vi "To Binary.vi"(8 "error in (no error)":errorcluster, 9 "byte order":T1(ring), 10 "Binary In":string, 11 "Double Float in":refnum<class "AbsFunc_One Term_DBL.lvclass">) -> (0 "error out":errorcluster, 2 "Binary":string, 3 "Double Float out":refnum<class "AbsFunc_One Term_DBL.lvclass">)   [LabVIEW 2021, in "AbsFunc_One Term_DBL.lvclass"]
uses:
  AbsFunc_One Term_DBL.lvclass
  AbsFunc_One Term_DBL.lvclass/AbsFunc_One Term_DBL.ctl
  Abs_Types/Double Float/Abs_Double Float.lvclass
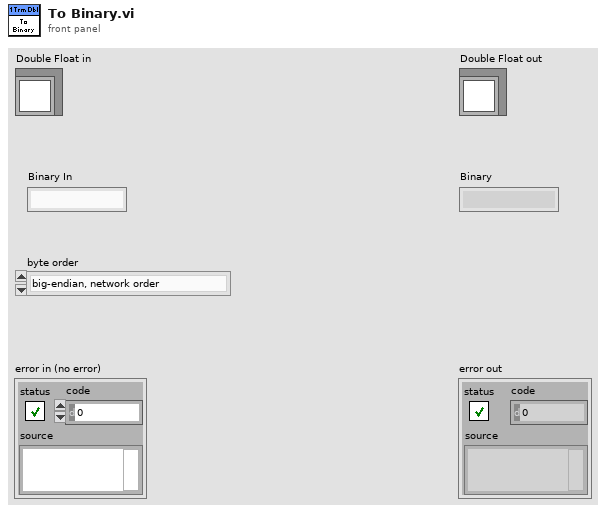
[diagram p1: front panel]
types:
  T1 = enum16{"big-endian, network order", "native, host order", "little-endian"}
  T2 = typedef "One Term_DBL.lvclass/Abstract Type.ctl" = refnum<class "Abs_Double Float.lvclass">
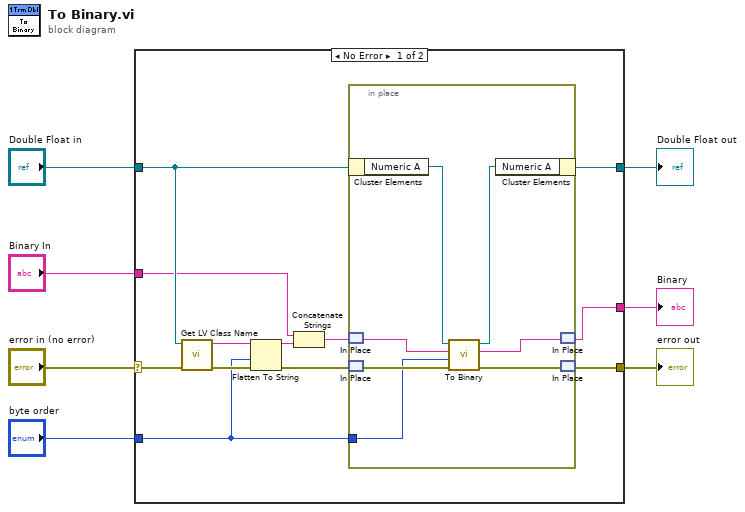
[diagram p0: block diagram]
diagram:
  n1 = case shown="No Error" "error in (no error)" {
    selector: "error in (no error)" -> [w19 w27]
    tunnel: "Binary In" -> [w10 w28]
    tunnel: "Double Float in" -> [w18 w29]
    tunnel: "byte order" -> [w12 _]
    tunnel: [w17 w27] -> w3
    tunnel: [w16 w28] -> w2
    tunnel: [w15 w29] -> w1
    frame No Error {
      n2 = call <vilib>:"Get LV Class Name.vi"("error in (no error)"=w19, "object"=w18) -> ("error out"=w13:errorcluster, "class name"=w14:string)  [unwired: 8 in]
      n3 = Flatten To String(anything=w14, byte order (0:big-endian, network order)=w12, error in (no error)=w13) -> (data string=w11:string, error out=w8:errorcluster)  [unwired: 1 in, 1 out]
      n4 = Concatenate Strings(w10, w11) -> (w9:string)
      n5 = in-place {
        in-place-border: w12 -> [w21]
        n6 = in-place-cluster #1(w18) -> ("Numeric A"=w26:T2)
        n7 = in-place-match #2(w9) -> (w24:string)
        n8 = in-place-match #3(w8) -> (w22:errorcluster)
        n9 = call-dynamic "To Binary.vi"("error in (no error)"=w22, "byte order"=w21, "Binary In"=w24, "Double Float in"=w26) -> ("error out"=w20:errorcluster, "Binary"=w23:string, "Double Float out"=w25:T2)  [unwired: 5 in]
        n10 = in-place-cluster #1("Numeric A"=w25) -> (w15:refnum<class "AbsFunc_One Term_DBL.lvclass">)
        n11 = in-place-match #2(w23) -> (w16:string)
        n12 = in-place-match #3(w20) -> (w17:errorcluster)
      }
    }
    frame Error {
    }
  }
  "error out" <- w3
  "Double Float out" <- w1
  "Binary" <- w2
